vi "Equation Explorer.vi"() -> ()   [LabVIEW 2023]
doc: "Demonstrates how to find the roots, or zeroes, for several equations that have several variables."
uses:
  <vilib>/gmath/zero.llb/nD Nonlinear System Solver (Formula).vi
  <vilib>/gmath/NI_Gmath.lvlib
panel:
  in  "Zeros":bool
  in  "Stop":bool
  in  "Chosen Zero":u16(ring) items=["0", "1", "2"]
  in  "End":dbl[](array[numeric])=[2.0, 2.0, 2.0, 2.0]
  in  "Number of Trials":u32=12
  in  "F(X)":string[](array[string])=["x+y+z-3+cos(x*y)", "x-y+z-1+x*y*z", "x-y-z+1-a", "cos(a+x-y)"]
  in  "X":string[](array[string])=["x", "y", "z", "a"]
  out "Zero":dbl[](array[numeric])
  out "F(zero)":dbl[](array[numeric])
  in  "Start":dbl[](array[numeric])=[0.0, 0.0, 0.0, 1.0]
  # "Overview: Demonstrates the use of the nD Nonlinear System Solver VI.\nRequirements: LabVIEW Full Development System\nInstructions: \n1. Run the VI. \n2. Click Zeros.\n3. Specify the index in Chosen Zero.\n4. Observe the values of Zero and F(zero).\n5. Click Stop to stop the VI."
  # "= 0"
  # "Note: After any calculation you have to choose the zeroes. There can be more than one solution."
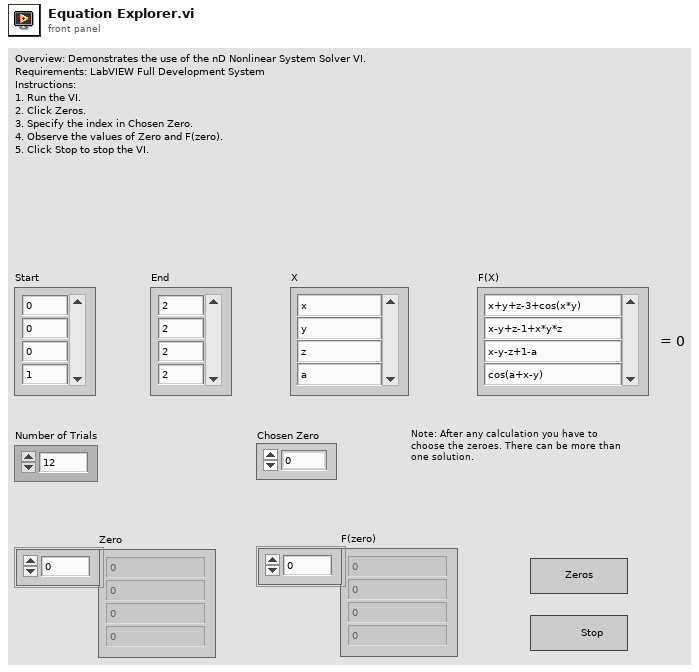
[diagram p1: front panel]
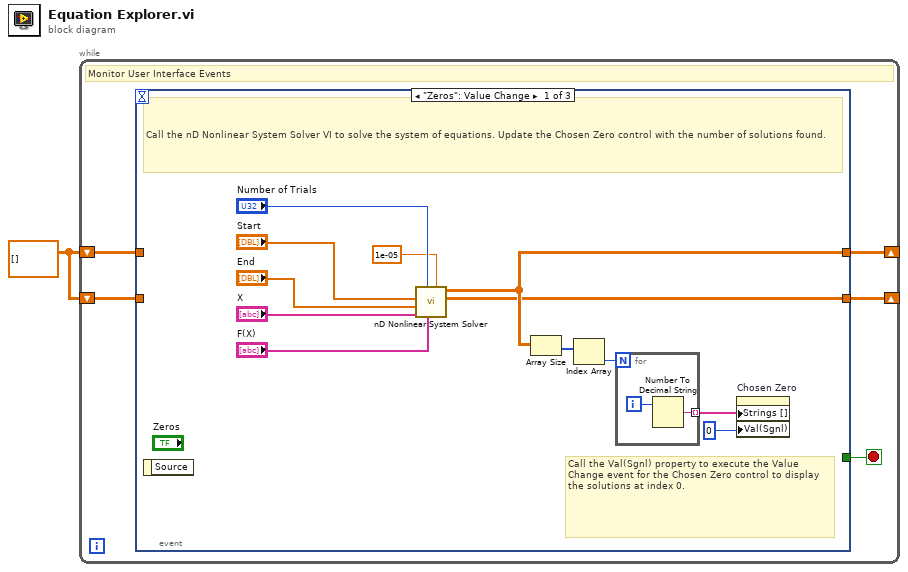
[diagram p0: block diagram]
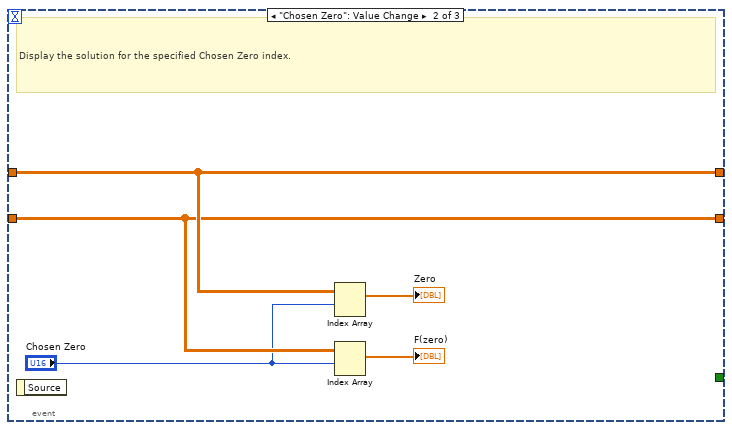
[diagram p2: hidden frame]
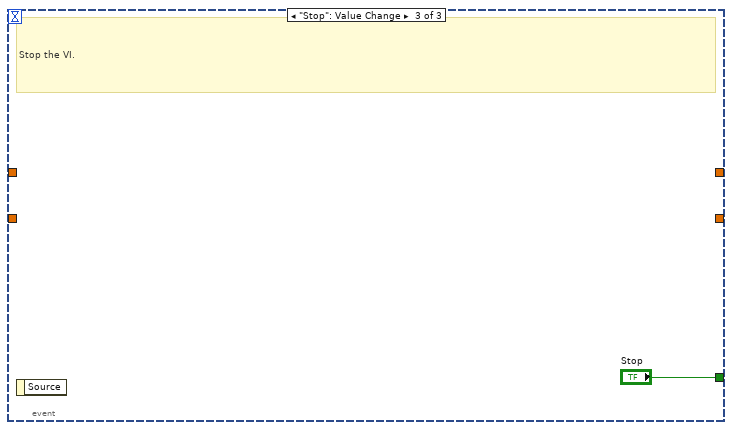
[diagram p3: hidden frame]
diagram:
  w1 = dbl[][] [] ("Zeroes")
  n1 = while {
    shift-left: w1 -> [w4]
    shift-right: [w5] -> _
    shift-left: w1 -> [w3]
    shift-right: [w6] -> _
    stop <- w2 stop-if-true
    # "Monitor User Interface Events"
    n2 = event shown="[0] \"Zeros\": Value Change" {
      selector: _ -> [_ _ _]
      dyn-events: _ -> [_ _ _]
      timeout: _ -> [_ _ _]
      tunnel: [w11 w25 _] -> w6
      tunnel: [w10 w24 _] -> w5
      tunnel: w4 -> [_ w24 _]
      tunnel: w3 -> [_ w25 _]
      tunnel: [_ _ "Stop"] -> w2
      event "Zeros": Value Change {
        # "Call the Val(Sgnl) property to execute the Value Change event for the Chosen Zero control to display the solutions at index 0."
        # "Call the nD Nonlinear System Solver VI to solve the system of equations. Update the Chosen Zero control with the number of solutions found."
        n3 = event-data() -> ()  [unwired: 1 in, 1 out]
        n4 = call-poly <vilib>:"nD Nonlinear System Solver.vi"("accuracy"=1e-05, "F(X)"="F(X)", "number of trials"="Number of Trials", "X"="X", "End"="End", "Start"="Start") -> ("f(Zeroes)"=w10:dbl[][], "Zeroes"=w11:dbl[][])  [unwired: 2 in, 2 out]
        n5 = Array Size(array=w11) -> (size(s)=w13:i32[])
        n6 = Index Array(array=w13) -> (element=w12:i32)  [unwired: 1 in]
        n7 = for {
          N: w12 -> [_]
          tunnel: [w20] -> w9 mode=indexing
          i -> [w19]
          n8 = Number To Decimal String(number=w19) -> (decimal integer string=w20:string)  [unwired: 1 in]
        }
        n9 = property on="Chosen Zero" class="Ring (strict)"("Strings []"=w9, "Val(Sgnl)"=0) -> ()  [unwired: 2 in, 2 out]
      }
      event "Chosen Zero": Value Change {
        # "Display the solution for the specified Chosen Zero index."
        n10 = event-data() -> ()  [unwired: 1 in, 1 out]
        n11 = Index Array(array=w25, index (row)="Chosen Zero") -> (element=→"Zero":dbl[])  [unwired: 1 in]
        n12 = Index Array(array=w24, index (row)="Chosen Zero") -> (element=→"F(zero)":dbl[])  [unwired: 1 in]
      }
      event "Stop": Value Change {
        # "Stop the VI."
        n13 = event-data() -> ()  [unwired: 1 in, 1 out]
      }
    }
  }
